vi "Build Channel Cluster Array.vi"() -> (3 "Channels out":cluster{"Channels":T1[]})   [LabVIEW 2023, in "Climate Chamber Cluster - 1 Channel.lvclass"]
uses:
  Climate Chamber Cluster - 1 Channel.lvclass
  Utilities/Channel.ctl
  Climate Chamber Cluster - 1 Channel.lvclass/Climate Chamber Cluster - 1 Channel.ctl
  Utilities/Utilities.lvlib
panel:
  in  "Channels in":cluster{"Channels":T1[]}
  in  "Chiller Cluster - 1 Channel.lvclass":refnum<class "Climate Chamber Cluster - 1 Channel.lvclass">
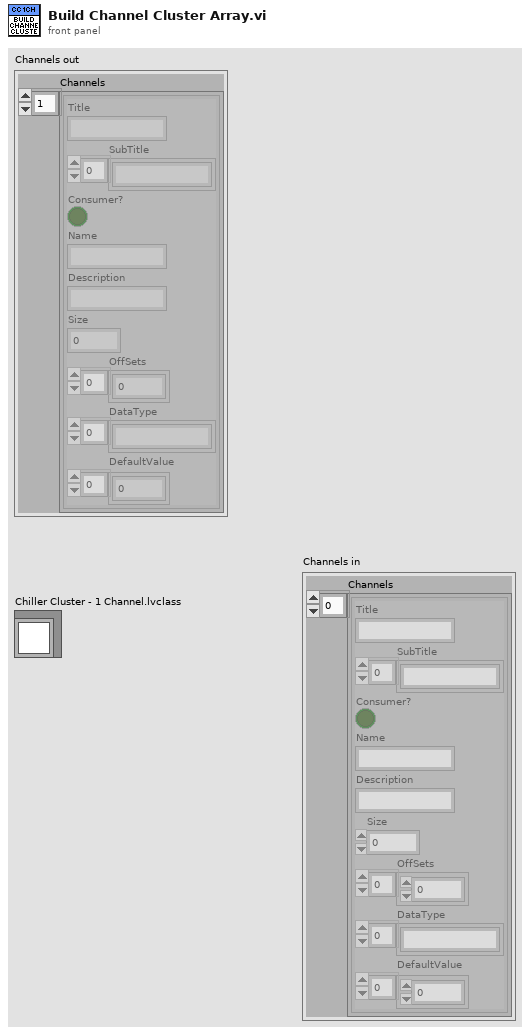
[diagram p1: front panel]
types:
  T1 = typedef "Utilities.lvlib/Channel.ctl" = cluster{"Title":string, "SubTitle":string[], "Consumer?":bool, "Name":string, "Description":string, "Size":i32, "OffSets":i32[], "DataType":string[], "DefaultValue":dbl[]}
  T2 = cluster{"OnOff.ACT":bool, "ErrorAcknowledge.ACT":bool}
  T3 = cluster{"OnOff.STS":i32, "Error.STS":i32, "Watchdog.STS":i32}
  T4 = cluster{"Temperature.ch01.SP":dbl, "TemperatureMIN.ch01.SP":dbl, "TemperatureMAX.ch01.SP":dbl, "TemperatureGrad.ch01.SP":dbl, "Humidity.ch01.SP":dbl, "HumidityMIN.ch01.SP":dbl, "HumidityMAX.ch01.SP":dbl, "HumidityGrad.ch01.SP":dbl}
  T5 = cluster{"Temperature.ch01.AV":dbl, "Humidity.ch01.AV":dbl}
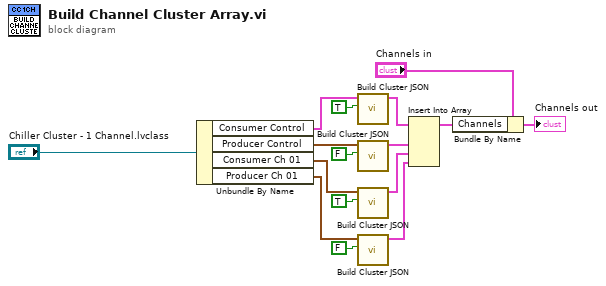
[diagram p0: block diagram]
diagram:
  n1 = Unbundle By Name("Chiller Cluster - 1 Channel.lvclass") -> ("Consumer Control"=w15:T2, "Producer Control"=w14:T3, "Consumer Ch 01"=w3:T4, "Producer Ch 01"=w4:T5)
  n2 = call "Build Cluster JSON.vi"("Consumer?"=TRUE, "Cluster"=w15) -> ("Array"=w11:T1[])  [unwired: 9 in]
  n3 = call "Build Cluster JSON.vi"("Consumer?"=FALSE, "Cluster"=w14) -> ("Array"=w10:T1[])  [unwired: 9 in]
  n4 = call "Build Cluster JSON.vi"("Consumer?"=TRUE, "Cluster"=w3) -> ("Array"=w2:T1[])  [unwired: 9 in]
  n5 = call "Build Cluster JSON.vi"("Consumer?"=FALSE, "Cluster"=w4) -> ("Array"=w1:T1[])  [unwired: 9 in]
  n6 = Insert Into Array(array=w11, new element #1=w10, new element #2=w2, new element #3=w1) -> (w8:T1[])  [unwired: 1 in]
  n7 = Bundle By Name(cluster="Channels in", "Channels"=w8) -> (→"Channels out":cluster{"Channels":T1[]})
